vi "top_vending.vi"() -> ()   [LabVIEW 2014]
panel:
  in  "Cluster":T1
  # "Piano Simulator"
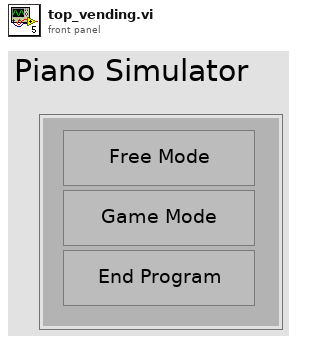
[diagram p1: front panel]
types:
  T1 = cluster{"Free mode":bool, "Game mode":bool, "Exit":bool}
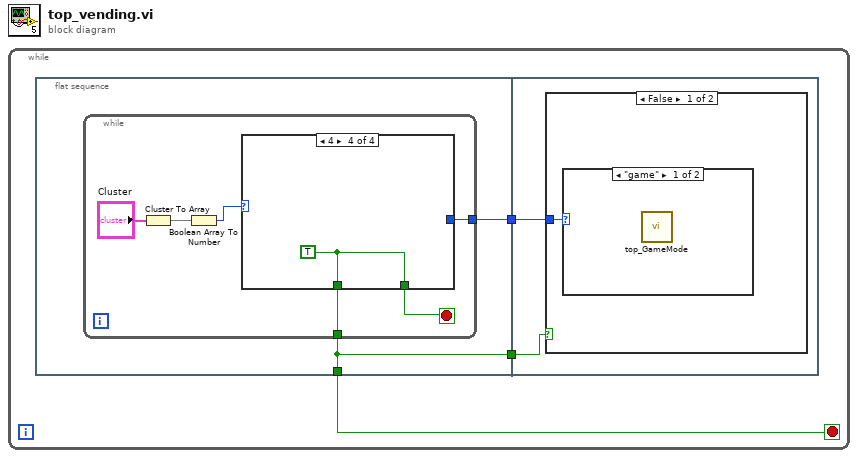
[diagram p0: block diagram]
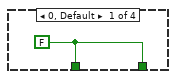
[diagram p2: hidden frame]
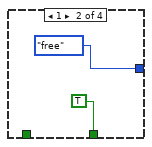
[diagram p3: hidden frame]
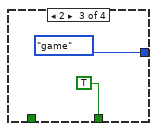
[diagram p4: hidden frame]
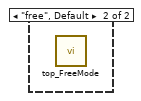
[diagram p5: hidden frame]
diagram:
  n1 = while {
    stop <- w2 stop-if-true
    n2 = flat-sequence {
      tunnel: [w5] -> w3
      tunnel: [w4] -> w2
      tunnel: [w4] -> w1
      tunnel: w3 -> [w19]
      tunnel: w1 -> [w18]
      frame #0 {
        n3 = while {
          tunnel: [w7] -> w5
          tunnel: [w6] -> w4
          stop <- w8 stop-if-true
          n4 = Cluster To Array(cluster="Cluster") -> (array=w10:bool[])
          n5 = Boolean Array To Number(Boolean array=w10) -> (number=w9:u32)
          n6 = case shown="4" w9 {
            tunnel: [w12 TRUE TRUE w17] -> w8
            tunnel: [_ enum16{"game", "free"}."free" enum16{"game", "free"}."game" _] -> w7
            tunnel: [w12 _ _ w17] -> w6
            frame 0, Default {
              w12 = FALSE
            }
            frame 1 {
            }
            frame 2 {
            }
            frame 4 {
              w17 = TRUE
            }
          }
        }
      }
      frame #1 {
        n7 = case shown="False" w18 {
          tunnel: w19 -> [w20 _]
          frame False {
            n8 = case shown="\"game\"" w20 {
              frame "game" {
                n9 = call "top_GameMode.vi"() -> ()  [unwired: 12 in]
              }
              frame "free", Default {
                n10 = call "top_FreeMode.vi"() -> ()  [unwired: 5 in, 2 out]
              }
            }
          }
          frame True {
          }
        }
      }
    }
  }
